vi "PH_SHS_Analysis.destructor.vi"(0 "i ref in":refnum<vi>, 5 "error in(no error)":errorcluster) -> (19 "error out":errorcluster)   [LabVIEW 2014, in "PH_SHS_Analysis.lvlib"]
doc: "This is the destructor of a class.\n\nLicense Agreement for this software:\n\nCopyright (C)\nGesellschaft für Schwerionenforschung, GSI\nPlanckstr. 1\n64291 Darmstadt\nGermany\n\nContact: D.Beck@gsi.de \n\nThis program is free software; you can redistribute it and/or modify it under the terms of the \nGNU General Public License as published by the Free Software Foundation; either version 2 of \nthe license, or (at your option) any later version.\n\nThis program is distributed in the hope that it will be useful, but WITHOUT ANY WARRANTY; \nwithout even the implied warranty of MERCHANTABILITY or FITNESS FOR A PARTICULAR PURPOSE. See the GNU General License for more details (http://www.gnu.org).\n\nGesellschaft für Schwerionenforschung, GSI\nPlanckstr. 1, 64291 Darmstadt, Germany\nFor all questions and ideas contact: M.Richter@gsi.de, H.Brand@gsi.de or D.Beck@gsi.de.\nLast update: 16-JUN-2004"
uses:
  PH_SHS_Analysis.lvlib
  PH_Basics/PH_Img_BaseClass/PH_Img_BaseClass.lvlib
  PH_Basics/PH_PSDBWriter/PH_PSDBWriter.lvlib
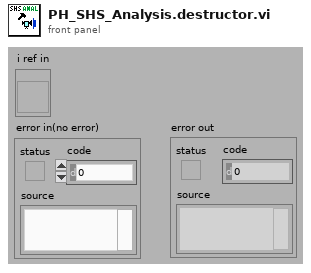
[diagram p1: front panel]
types:
  T1 = enum16{"SetAttribute", "GetAttribute", "CreateAttribute", "DestroyAttribute", "DestroyAllAtributes"}
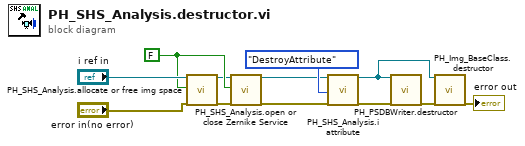
[diagram p0: block diagram]
diagram:
  w5 = FALSE ("Allocate?")
  n1 = call "PH_SHS_Analysis.allocate or free img space.vi"("i ref in"="i ref in", "Allocate?"=w5, "error in (no error)"="error in(no error)") -> ("i ref out"=w4:refnum<vi>, "error out"=w6:errorcluster)  [unwired: 15 in]
  n2 = call "PH_SHS_Analysis.open or close Zernike Service.vi"("i ref in"=w4, "open"=w5, "error in (no error)"=w6) -> ("i ref out"=w2:refnum<vi>, "error out"=w3:errorcluster)  [unwired: 15 in]
  n3 = call "PH_SHS_Analysis.i attribute.vi"("VI Refnum"=w2, "Action"=T1."DestroyAttribute", "error in (no error)"=w3) -> ("VI Refnum out"=w1:refnum<vi>, "error out"=w11:errorcluster)  [unwired: 14 in, 1 out]
  n4 = call "PH_PSDBWriter.destructor.vi"("i ref in"=w1, "error in(no error)"=w11) -> ("error out"=w10:errorcluster)  [unwired: 17 in]
  n5 = call "PH_Img_BaseClass.destructor.vi"("i ref in"=w1, "error in(no error)"=w10) -> ("error out"=→"error out":errorcluster)  [unwired: 17 in]
